vi "Colour Items of a JSON string control.vi"(6 "Defer Panel Updates":bool, 7 "Maximum UI Property calls":i32=-1, 8 "error in (no error)":errorcluster, 10 "String Control":refnum<vi>, 11 "JSON":string) -> (0 "error out":errorcluster)   [LabVIEW 2019, in "JSONtext.lvlib"]
doc: "Writes the input JSON to a string control and colour the elements for better readability. Note that this may be slow for large JSON structures; consider the following options\"\n1) Defer Panel Updates set to true will speed up the process by preventing display redraws untill all items are coloured. \n2) You may set a limit to number of elements that are actually coloured in order to ensure the VI completes in a reasonable amount of time (the default of -1 means no limit)."
uses:
  JSONtext.lvlib
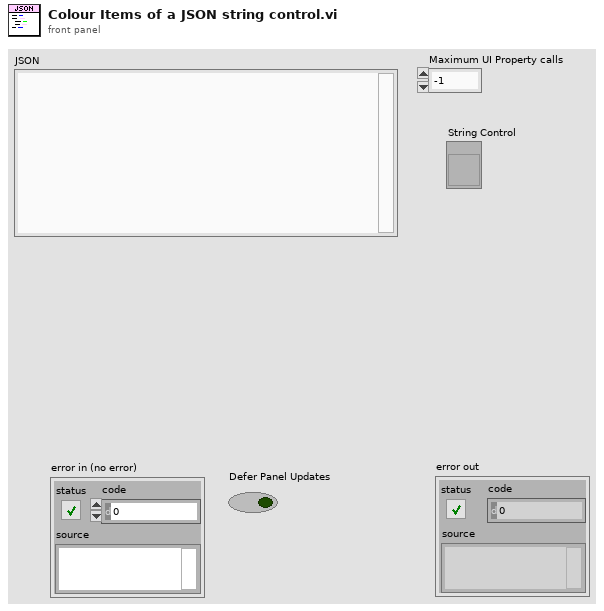
[diagram p1: front panel]
types:
  T1 = typedef "JSONtext.lvlib/JSON Value Type.ctl" = enum16{"Not a JSON Value", "JSON Object", "JSON Array", "String", "Number", "true", "false", "null"}
  T2 = cluster{"Value start out":i32, "Offset past match":i32, "JSON Value Type":T1}[]
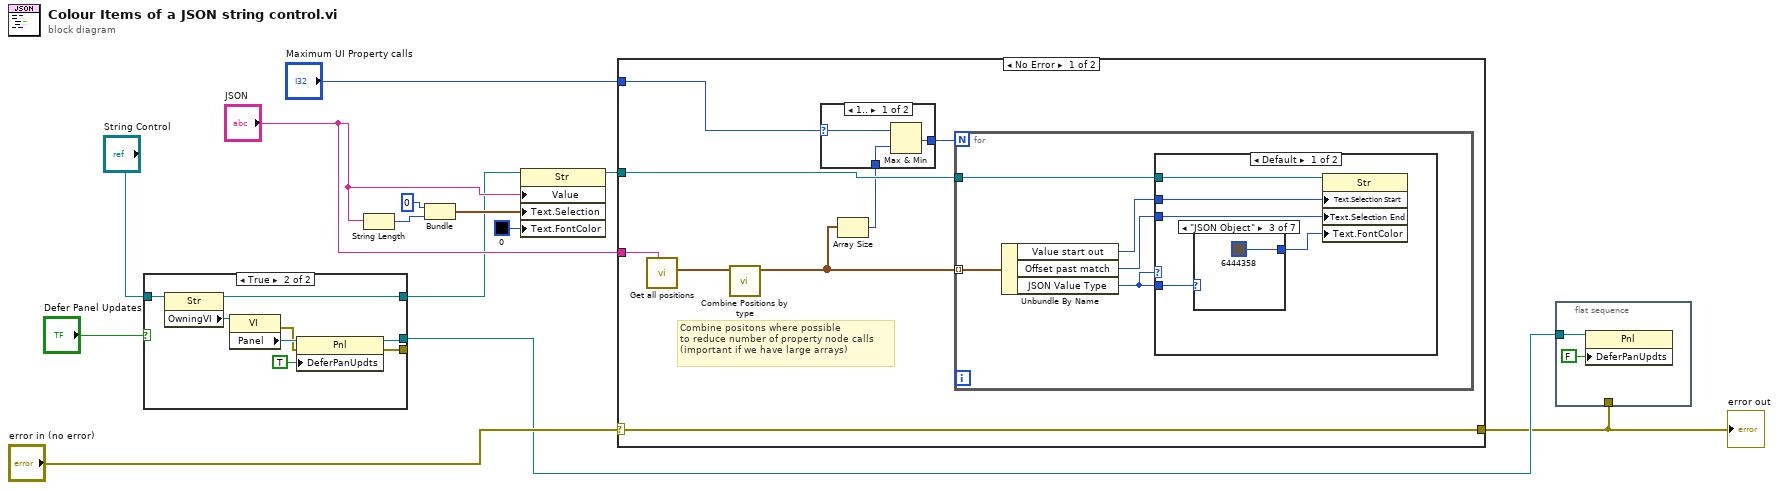
[diagram p0: block diagram]
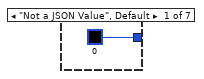
[diagram p4: hidden frame]
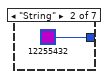
[diagram p5: hidden frame]
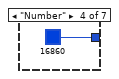
[diagram p6: hidden frame]
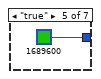
[diagram p7: hidden frame]
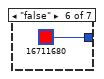
[diagram p8: hidden frame]
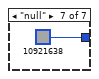
[diagram p9: hidden frame]
diagram:
  n1 = case shown="True" "Defer Panel Updates" {
    tunnel: "String Control" -> [w14 w22]
    tunnel: [w14 w21] -> w4
    tunnel: [_ w16] -> w2
    tunnel: [_ w15] -> _
    frame False {
    }
    frame True {
      n2 = property class="Str"(reference=w22) -> (reference out=w21:refnum<vi>, "OwningVI"=w20:refnum<vi>)  [unwired: 1 in, 1 out]
      n3 = property class="VI"(reference=w20) -> (error out=w17:errorcluster, "Panel"=w18:refnum<vi>)  [unwired: 1 in, 1 out]
      n4 = property class="Pnl"(reference=w18, error in=w17, "DeferPanUpdts"=TRUE ("Defer Panel Updates")) -> (reference out=w16:refnum<vi>, error out=w15:errorcluster)
    }
  }
  n5 = String Length(string="JSON") -> (length=w12:i32)
  n6 = Bundle("Selection Start"=u32 0, w12) -> (w11:cluster{"Selection Start":u32, i32})  [unwired: 1 in]
  n7 = property on="Property Node" class="Str"(reference=w4, "Value"="JSON", "Text.Selection"=w11, "Text.FontColor"=u32 0) -> (reference out=w9:refnum<vi>)  [unwired: 1 in, 1 out]
  n8 = case shown="No Error" "error in (no error)" {
    selector: "error in (no error)" -> [w23 w52]
    tunnel: w9 -> [w30 _]
    tunnel: "JSON" -> [w29 _]
    tunnel: "Maximum UI Property calls" -> [w26 _]
    tunnel: [w23 w52] -> w1
    frame No Error {
      # "Combine positons where possible \nto reduce number of property node calls\n(important if we have large arrays)"
      n9 = call "Get all positions.vi"("JSON"=w29) -> ("Array"=w28:T2)  [unwired: 8 in, 2 out]
      n10 = call "Combine Positions by type.vi"("Array in"=w28) -> ("Array out"=w25:T2)  [unwired: 10 in]
      n11 = Array Size(array=w25) -> (size(s)=w24:i32)
      n12 = case shown="1.." w26 {
        selector: w26 -> [w31 _]
        tunnel: [w33 w34] -> w27
        tunnel: w24 -> [w32 w34]
        frame 1.. {
          n13 = Max & Min(x=w31, y=w32) -> (min(x,y)=w33:i32)  [unwired: 1 out]
        }
        frame ..0 {
        }
      }
      n14 = for {
        N: w27 -> [_]
        tunnel: w25 -> [w39] mode=indexing
        tunnel: w30 -> [w35]
        n15 = Unbundle By Name(w39) -> ("Value start out"=w38:i32, "Offset past match"=w37:i32, "JSON Value Type"=w36:T1)
        n16 = case shown="Default" w36 {
          tunnel: w36 -> [w44 _]
          tunnel: w38 -> [w42 _]
          tunnel: w37 -> [w41 _]
          tunnel: w35 -> [w40 _]
          frame Default {
            n17 = case shown="\"JSON Object\"" w44 {
              tunnel: [u32 0 u32 12255432 u32 6444358 u32 16860 u32 1689600 u32 16711680 u32 10921638] -> w43
              frame "Not a JSON Value", Default {
              }
              frame "String" {
              }
              frame "JSON Object" {
              }
              frame "Number" {
              }
              frame "true" {
              }
              frame "false" {
              }
              frame "null" {
              }
            }
            n18 = property on="Property Node" class="Str"(reference=w40, "Text.Selection Start"=w42, "Text.Selection End"=w41, "Text.FontColor"=w43) -> ()  [unwired: 1 in, 2 out]
          }
          frame "JSON Object" {
          }
        }
      }
    }
    frame Error {
    }
  }
  "error out" <- w1
  n19 = flat-sequence {
    tunnel: w2 -> [w53]
    tunnel: w1 -> [_]
    frame #0 {
      n20 = property class="Pnl"(reference=w53, "DeferPanUpdts"=FALSE ("Defer Panel Updates")) -> ()  [unwired: 1 in, 2 out]
    }
  }
